vi "mergeVISAPropNode.vi"   [LabVIEW 2017]
doc: "Gets (reads) and/or sets (writes) properties of a reference. The node operates in the same way as a standard Property Node."
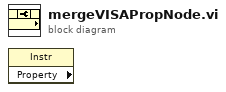
[diagram p0: block diagram]
diagram:
  n1 = property class="Instr" props=[]() -> ()  [unwired: 2 in, 3 out]
